vi "Write Server Internal UEs.vi"(8 "error in (no error)":errorcluster, 10 "Server Internal UEs":T1, 11 "gRPC service in":refnum<class "Template.lvclass">) -> (0 "error out":errorcluster, 3 "gRPC service out":refnum<class "Template.lvclass">)   [LabVIEW 2021, in "Template_server.lvlib" / "Template.lvclass"]
uses:
  Template.lvclass
  typeDefs/Server Internal UEs.ctl
  typeDefs/Server Internal Message.ctl
  Template.lvclass/Template.ctl
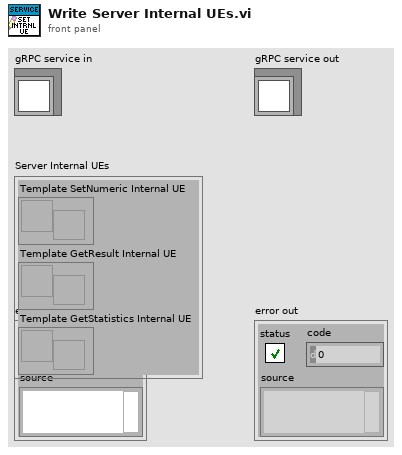
[diagram p1: front panel]
types:
  T1 = typedef "Template_server.lvlib/Template.lvclass/Server Internal UEs.ctl" = cluster{"Template SetNumeric Internal UE":refnum<user-event>, "Template GetResult Internal UE":refnum<user-event>, "Template GetStatistics Internal UE":refnum<user-event>}
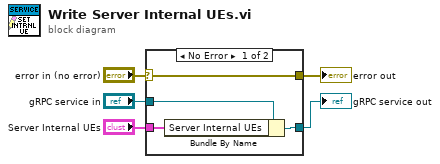
[diagram p0: block diagram]
diagram:
  n1 = case shown="No Error" "error in (no error)" {
    selector: "error in (no error)" -> [w9 w10]
    tunnel: [w9 w10] -> w4
    tunnel: [w7 w11] -> w2
    tunnel: "gRPC service in" -> [w8 w11]
    tunnel: "Server Internal UEs" -> [w6 _]
    frame No Error {
      n2 = Bundle By Name(cluster=w8, "Server Internal UEs"=w6) -> (w7:refnum<class "Template.lvclass">)
    }
    frame Error {
    }
  }
  "error out" <- w4
  "gRPC service out" <- w2
